vi "Build 110 130 Array.vi"(8 "Error In":errorcluster, 11 "Filtered Array":string[][](array[string])) -> (0 "Error Out":errorcluster, 3 "110-130 Array":dbl[][](array[numeric]))   [LabVIEW 2019]
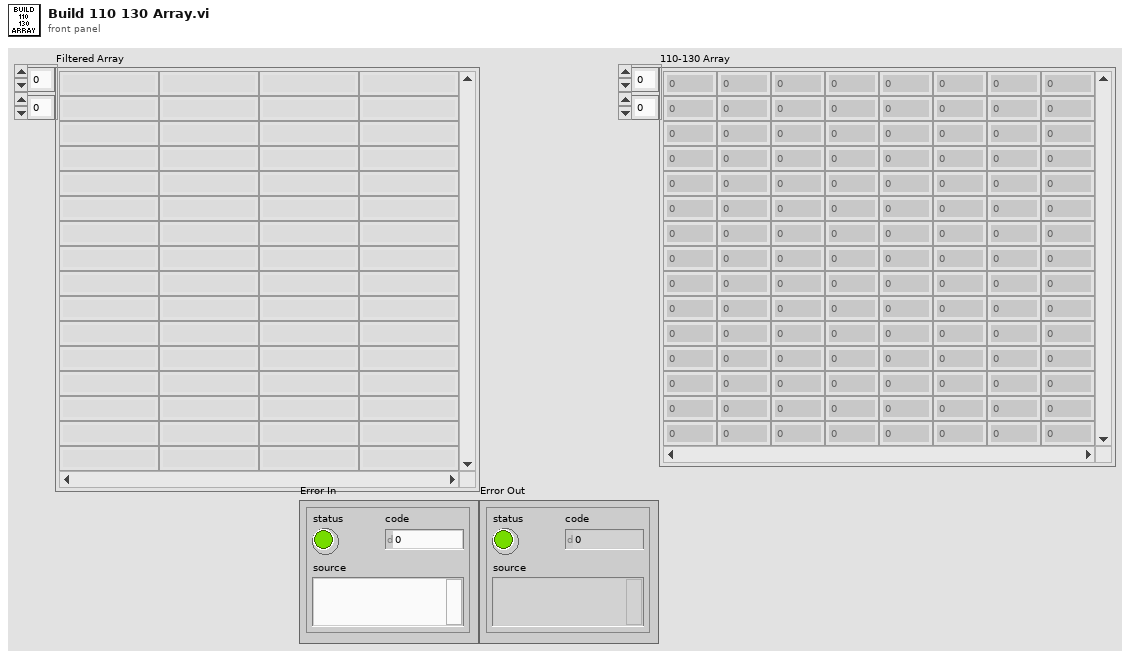
[diagram p1: front panel]
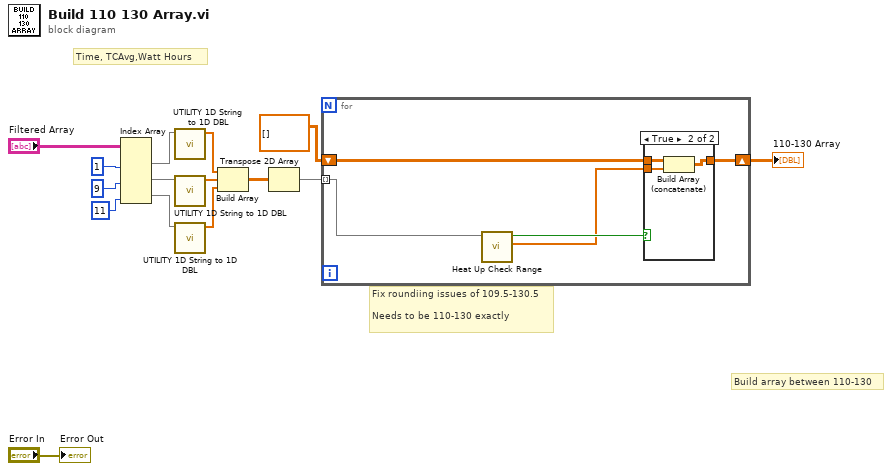
[diagram p0: block diagram]
diagram:
  # "Fix roundiing issues of 109.5-130.5\n\nNeeds to be 110-130 exactly"
  # "Build array between 110-130"
  # "Time, TCAvg,Watt Hours"
  n1 = Index Array(array="Filtered Array", index (col) #1=1 ("disabled index (col)"), index (col) #2=9 ("index (col)"), index (col) #3=11 ("index (col)")) -> (element #1=w5:string[], element #2=w6:string[], element #3=w7:string[])  [unwired: 3 in]
  n2 = call "UTILITY 1D String to 1D DBL.vi"("Save Data"=w5) -> ("DBL"=w12:dbl[])  [unwired: 10 in]
  n3 = call "UTILITY 1D String to 1D DBL.vi"("Save Data"=w6) -> ("DBL"=w11:dbl[])  [unwired: 10 in]
  n4 = call "UTILITY 1D String to 1D DBL.vi"("Save Data"=w7) -> ("DBL"=w13:dbl[])  [unwired: 10 in]
  n5 = Build Array(w12, w11, w13) -> (w8:dbl[][])
  n6 = Transpose 2D Array(2D array=w8) -> (transposed array=w9:dbl[][])
  n7 = for {
    tunnel: w9 -> [w17] mode=indexing
    shift-right: [w19] -> w14
    shift-left: dbl[][] [] -> [w20]
    n8 = call "Heat Up Check Range.vi"("Array"=w17) -> ("Ouput Data"=w16:dbl[], "Add This Row"=w18:bool)  [unwired: 9 in]
    n9 = case shown="True" w18 {
      tunnel: w20 -> [w21 w24]
      tunnel: [w21 w23] -> w19
      tunnel: w16 -> [_ w22]
      frame False {
      }
      frame True {
        n10 = Build Array (concatenate)(w24, w22) -> (w23:dbl[][])
      }
    }
  }
  "110-130 Array" <- w14
  "Error Out" <- "Error In"
